vi "Autonomous Independent.vi"() -> ()   [LabVIEW 2011]
doc: "This VI is called when autonomous begins, and will automatically be terminated when autonomous ends. You can carry out timed or sensor driven robot movement independently without needing to return to the caller."
uses:
  Robot Global Data.vi
  <vilib>/Rock Robotics/WPI/RobotDrive/WPI_RobotDriveArcadeDrive_Standard(NoSaturation).vi
panel:
  in  "Limit Switch Placeholder":bool
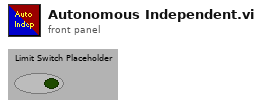
[diagram p1: front panel]
types:
  T1 = typedef "WPI_JoystickDevRef.ctl" = cluster{"Device":T2}
  T2 = typedef "WPI_JoystickDeviceEnum.ctl" = enum16{"USB 1", "USB 2", "USB 3", "USB 4", "Kinect 1", "Kinect 2"}
  T3 = typedef "WPI_RelayDevRef.ctl" = cluster{"DevStatus":errorcluster, "Relay Channel":T4, "Digital Module":T5, "Relay Direction":T6}
  T4 = typedef "FPGA_DIORelayChannel.ctl" = enum8{"Relay 1", "Relay 2", "Relay 3", "Relay 4", "Relay 5", "Relay 6", "Relay 7", "Relay 8", "Invalid"}
  T5 = typedef "FPGA_TypedefDigitalModule.ctl" = enum16{"Digital Module 1", "Digital Module 2"}
  T6 = typedef "WPI_RelayDirection.ctl" = enum16{"Both directions", "Forward only", "Reverse only"}
  T7 = typedef "WPI_RobotDriveDevRef.ctl" = cluster{"DevStatus":errorcluster, "Motors[]":T8[], "Square Inputs":bool, "Max Output":dbl, "Isochronous":bool}
  T8 = typedef "WPI_MotorControlDeviceRef.ctl" = cluster{"DeviceStatus":errorcluster, "Type":enum16{"PWM", "CAN"}, "PWM":cluster{"Digital Module":T5, "PWM Channel":T9, "DeadBand":T10}, "CAN":cluster{"Device Number":u8, "Control Mode":T11, "Semaphore":T12, "Max Vout":dbl}, "Invert":bool, "TransformRef":T13, "InvTransformRef":T13}
  T9 = typedef "FPGA_DIOPWMChannel.ctl" = enum8{"PWM 1", "PWM 2", "PWM 3", "PWM 4", "PWM 5", "PWM 6", "PWM 7", "PWM 8", "PWM 9", "PWM 10", "Invalid"}
  T10 = typedef "WPI_PWMDeadband.ctl" = cluster{"Name":string, "maxPositivePwm":i32, "minPositivePwm":i32, "centerPwm":i32, "maxNegativePwm":i32, "minNegativePwm":i32, "angularRange":u16}
  T11 = typedef "WPI_CANJaguar_ControlMode.ctl" = enum8{"Percent VBus", "Current", "Speed", "Position", "Voltage"}
  T12 = typedef "Semaphore RefNum" = refnum<k1>
  T13 = typedef "WPI_PWMTransform_ConPane.ctl" = refnum<vi>
  T14 = cluster{"axis 1 (x)":dbl, "axis 2 (y)":dbl, "axis 3 (throttle)":dbl, "axis 4":dbl, "axis 5":dbl, "axis 6":dbl}
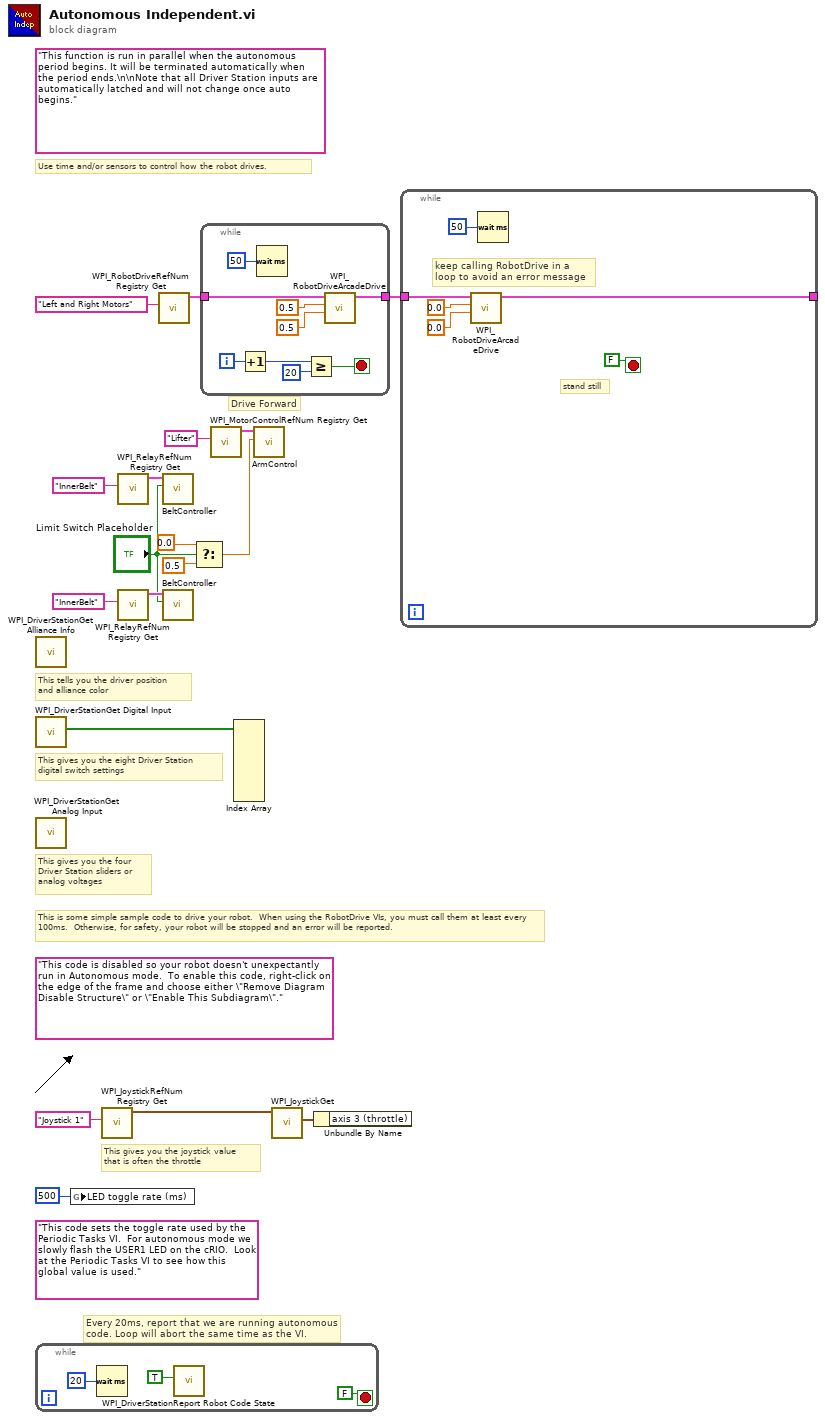
[diagram p0: block diagram]
diagram:
  (unwired) "This code sets the toggle rate used by the Periodic Tasks VI.  For autonomous mode we slowly flash the USER1 LED on the cRIO.  Look at the Periodic Tasks VI to see how this global value is used."
  (unwired) "This code is disabled so your robot doesn't unexpectantly run in Autonomous mode.  To enable this code, right-click on the edge of the frame and choose either \"Remove Diagram Disable Structure\" or \"Enable This Subdiagram\"."
  (unwired) "This function is run in parallel when the autonomous period begins. It will be terminated automatically when the period ends.\n\nNote that all Driver Station inputs are automatically latched and will not change once auto begins."
  # "This is some simple sample code to drive your robot.  When using the RobotDrive VIs, you must call them at least every 100ms.  Otherwise, for safety, your robot will be stopped and an error will be reported."
  # "stand still"
  # "Drive Forward"
  # "Every 20ms, report that we are running autonomous\ncode. Loop will abort the same time as the VI."
  # "This gives you the joystick value\nthat is often the throttle"
  # "Use time and/or sensors to control how the robot drives."
  # "This tells you the driver position\nand alliance color"
  # "This gives you the eight Driver Station\ndigital switch settings"
  # "This gives you the four\nDriver Station sliders or\nanalog voltages"
  n1 = call <vilib>:"WPI_DriverStationGet Alliance Info.vi"() -> ()  [unwired: 12 out]
  n2 = call <vilib>:"WPI_DriverStationGet Digital Input.vi"() -> ("Driver Station Digital Input (1-8)"=w18:bool[])  [unwired: 11 out]
  n3 = call <vilib>:"WPI_DriverStationGet Analog Input.vi"() -> ()  [unwired: 12 out]
  n4 = while {
    stop <- FALSE stop-if-true
    n5 = Wait (ms)(milliseconds to wait=u32 20) -> ()  [unwired: 1 out]
    n6 = call <vilib>:"WPI_DriverStationReport Robot Code State.vi"("Autonomous"=TRUE) -> ()  [unwired: 10 in, 1 out]
  }
  n7 = global write "Robot Global Data.vi" "LED toggle rate (ms)"(u32 500 ("LED ms toggle rate")) -> ()
  n8 = call <vilib>:"WPI_JoystickRefNum Registry Get.vi"("refnum name"="Joystick 1") -> ("JoystickDevRef"=w15:T1)  [unwired: 1 in, 9 out]
  n9 = call <vilib>:"WPI_RelayRefNum Registry Get.vi"("refnum name"="InnerBelt") -> ("RelayDevRef"=w9:T3)  [unwired: 9 in, 1 out]
  n10 = call <vilib>:"WPI_RelayRefNum Registry Get.vi"("refnum name"="InnerBelt") -> ("RelayDevRef"=w7:T3)  [unwired: 9 in, 1 out]
  n11 = call <vilib>:"WPI_RobotDriveRefNum Registry Get.vi"("refnum name"="Left and Right Motors") -> ("RobotDriveDevRef"=w12:T7)  [unwired: 1 in, 9 out]
  n12 = call "BeltController.vi"("Control Button"="Limit Switch Placeholder", "RelayDevRef"=w9) -> ()  [unwired: 10 in]
  n13 = call "BeltController.vi"("Control Button"="Limit Switch Placeholder", "RelayDevRef"=w7) -> ()  [unwired: 10 in]
  n14 = Select(t=0.0, s="Limit Switch Placeholder", f=0.5) -> (s? t:f=w4:dbl)
  n15 = while {
    tunnel: w12 -> [w30]
    tunnel: [w23] -> w11
    i -> [w26]
    stop <- w24 stop-if-true
    n16 = Increment(x=w26) -> (x+1=w22:i32)
    n17 = Wait (ms)(milliseconds to wait=u32 50) -> ()  [unwired: 1 out]
    n18 = Greater Or Equal?(x=w22, y=20) -> (x >= y?=w24:bool)
    n19 = call-poly <vilib>:"WPI_RobotDriveArcadeDrive.vi"("Y axis value"=0.5 ("X axis value"), "X axis value"=0.5, "RobotDriveDevRef"=w30) -> ("RobotDriveDevRef"=w23:T7)  [unwired: 1 in, 7 out]
  }
  n20 = call <vilib>:"WPI_MotorControlRefNum Registry Get.vi"("refnum name"="Lifter") -> ("MotorControlDevRef"=w5:T8)  [unwired: 9 in, 1 out]
  n21 = Index Array(array=w18) -> ()  [unwired: 8 in, 8 out]
  n22 = call "ArmControl.vi"("Speed"=w4, "MotorControlDevRef"=w5) -> ()  [unwired: 8 in]
  n23 = call <vilib>:"WPI_JoystickGet.vi"("JoystickDevRef"=w15) -> ("Axes"=w16:T14)  [unwired: 1 in, 5 out]
  n24 = Unbundle By Name(w16) -> ()  [unwired: 1 out]
  n25 = while {
    tunnel: w11 -> [w36]
    tunnel: [w32] -> _
    stop <- FALSE stop-if-true
    # "keep calling RobotDrive in a loop to avoid an error message"
    n26 = call-poly <vilib>:"WPI_RobotDriveArcadeDrive.vi"("Y axis value"=0.0 ("X axis value"), "X axis value"=0.0, "RobotDriveDevRef"=w36) -> ("RobotDriveDevRef"=w32:T7)  [unwired: 1 in, 7 out]
    n27 = Wait (ms)(milliseconds to wait=u32 50) -> ()  [unwired: 1 out]
  }
